vi "Write Event Data to File.vi"(8 "error in (no error)":errorcluster, 9 "Event Data String":string, 10 "Event String":string, 11 "File Operations":T1) -> (0 "error out":errorcluster)   [LabVIEW 8.6]
doc: "Performs File Functions for the Event Log\n\nOpen File opens the data log file or creates it if not found.\nWrite Log Data writes the supplied Event String and Event Data String to file along with the current timestamp.\nClose File closes the file reference."
uses:
  Controls/File Command Enum.ctl
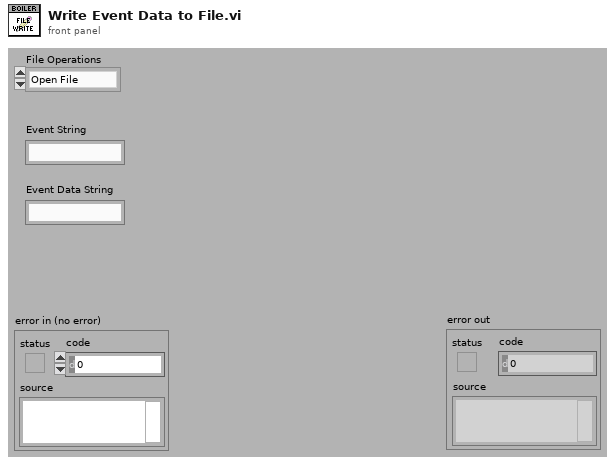
[diagram p1: front panel]
types:
  T1 = typedef "File Command Enum.ctl" = enum16{"Open File", "Write Log Data", "Close File"}
  T2 = enum16{"open", "replace", "create", "open or create", "replace or create", "replace or create with confirmation"}
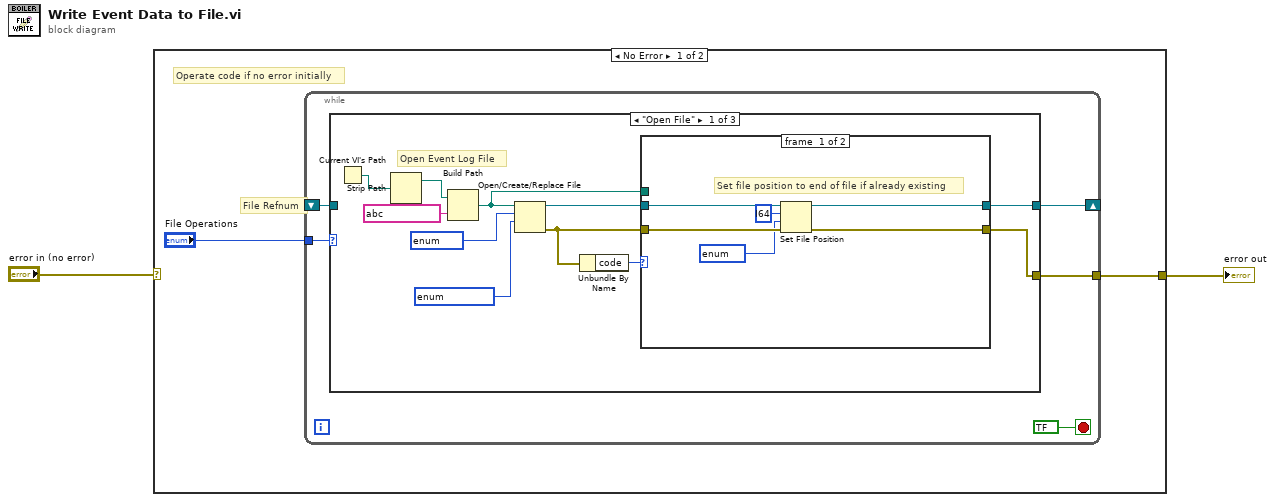
[diagram p0: block diagram]
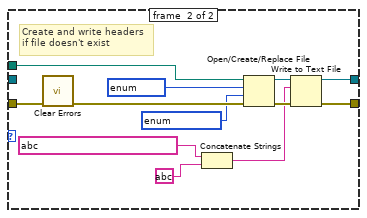
[diagram p2: hidden frame]
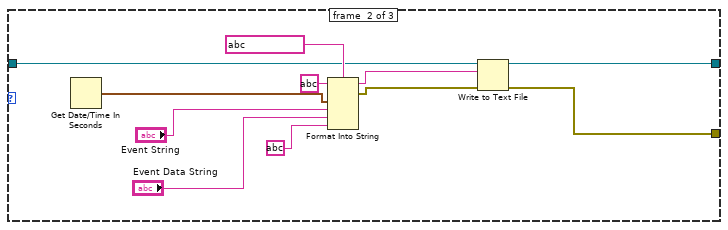
[diagram p3: hidden frame]
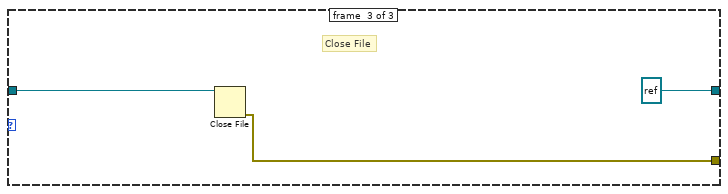
[diagram p4: hidden frame]
diagram:
  n1 = case shown="No Error" "error in (no error)" {
    selector: "error in (no error)" -> [_ w53]
    tunnel: [w3 w53] -> w1
    frame #0 {
      # "File Refnum"
      # "Operate code if no error initially"
      n2 = while {
        tunnel: "File Operations" -> [w8]
        shift-right: [w7] -> _
        shift-left: _ -> [w6]
        tunnel: [w5] -> w3
        stop <- bool ? stop-if-true
        n3 = case shown="\"Open File\"" w8 {
          tunnel: [w11 w41 refnum<file> ? ("refnum out")] -> w7
          tunnel: w6 -> [_ w44 w52]
          tunnel: [w10 w42 w51] -> w5
          frame #0 {
            # "Open Event Log File"
            n4 = Current VI's Path() -> (path=w20:path)
            n5 = Strip Path(path=w20) -> (stripped path=w19:path)  [unwired: 1 out]
            n6 = Build Path(base path=w19, name or relative path=string ?) -> (appended path=w13:path)
            n7 = Open/Create/Replace File(file path (use dialog)=w13, operation (0:open)=T2 ?, access (0:read/write)=enum16{"read/write", "read-only", "write-only"} ?) -> (refnum out=w12:refnum<file>, error out=w14:errorcluster)  [unwired: 3 in, 1 out]
            n8 = Unbundle By Name(w14) -> ("code"=w15:i32)
            n9 = case shown="7" w15 {
              tunnel: w14 -> [w25 w38]
              tunnel: w13 -> [_ w36]
              tunnel: [w23 w30] -> w10
              tunnel: [w24 w31] -> w11
              tunnel: w12 -> [w26 _]
              frame #0 {
                # "Set file position to end of file if already existing"
                n10 = Set File Position(offset (in bytes) (0)=i64 ?, refnum=w26, from (0:start)=enum16{"start", "end", "current"} ?, error in=w25) -> (refnum out=w24:refnum<file>, error out=w23:errorcluster)
              }
              frame #1 {
                # "Create and write headers\nif file doesn't exist"
                n11 = call <vilib>:"Clear Errors.vi"("error in (no error)"=w38) -> ("error out"=w37:errorcluster)  [unwired: 6 in]
                n12 = Concatenate Strings(string ?, string ?) -> (w27:string)
                n13 = Open/Create/Replace File(file path (use dialog)=w36, error in=w37, operation (0:open)=T2 ?, access (0:read/write)=enum16{"read/write", "read-only", "write-only"} ?) -> (refnum out=w33:refnum<file>, error out=w32:errorcluster)  [unwired: 2 in, 1 out]
                n14 = Write to Text File(file (use dialog)=w33, text=w27, error in=w32) -> (refnum out=w31:refnum<file>, error out=w30:errorcluster)  [unwired: 1 in, 1 out]
              }
            }
          }
          frame #1 {
            n15 = Get Date/Time In Seconds() -> (seconds since 1Jan1904=w48:timestamp)
            n16 = Format Into String(format string=string ?, initial string=string ?, w48, "Event String", "Event Data String", string ?) -> (resulting string=w40:string, error out=w43:errorcluster)  [unwired: 1 in]
            n17 = Write to Text File(file (use dialog)=w44, text=w40, error in=w43) -> (refnum out=w41:refnum<file>, error out=w42:errorcluster)  [unwired: 1 in, 1 out]
          }
          frame #2 {
            # "Close File"
            n18 = Close File(refnum=w52) -> (error out=w51:errorcluster)  [unwired: 1 in, 1 out]
          }
        }
      }
    }
    frame #1 {
      # "Pass error through if present on entry"
    }
  }
  "error out" <- w1
